vi "Demo File Dialog.vi"(8 "error in (no error)":errorcluster) -> (0 "error out":errorcluster)   [LabVIEW 2011]
uses:
  VIremote.llb/VIremoteEvent.ctl
  VIremote.llb/VIremoteFunction.ctl
panel:
  out "Selected File":path
  in  "Browse":bool
  in  "Select File":i32(ring)=1 items=["-C:\\_ics_ab\\dev\\vi.lib\\Throw Lab\\VIremote\\Examples", "Parent Folder", "-Folders", "server", "-Files", "All_Demos.vi", "Demo Accelerometer Graph.vi", "Demo Button and Alert server.vi", "Demo Button and Alert.vi", "Demo Combo Box.vi", "Demo Date and Time.vi", "Demo Dialog.vi", "Demo File Dialog.vi", "Demo Input Advanced.vi", "Demo Multitouch.vi", "Demo Navigation Bar More.vi", "Demo Navigation Bar.vi", "Demo Play wav file to Sound Output.vi", "Demo Ring and Enum.vi", "Demo Scrolling.vi", "Demo Simple Sound.vi", "Demo Slider.vi", "Demo Sound File to Sound Output.vi", "Demo Sound Input Output.vi", "Demo Sound Input.vi", "Demo Sound Input2.vi", "Demo String and Numeric.vi", "Demo UI Orientation.vi", "Demo User Notification and Status.vi", "Demo Video Input.vi", "Demo Video Input2.vi", "Hello World.vi", "sample.wav", "Server_Demo.vi", "VIremoteDisplaySimulator.vi", "VIs_for_All_Demos.vi", "xxx.vi"]
  in  "VIremoteEvent":T1=enum."Connection Closed"
  # "This is an example of how you could make a File Dialog. The ring above should be hidden under the button or the Selected File indicator. The code in the \"Ring Value Change\" case could be placed in a separate \"select path\" VI.\n\nThe Description of the ring above is:\n\nVIREMOTEPROPERTIES\nStyle=Grouped\nHeight=600\nUpdateWhileChanging\n\nThe height is for the iPad popover so it won't try to adjust its size. 600 is a good value for a large popover in both landscape and portrait mode.\n\nUpdateWhileChanging will prevent the table view to close when an item is selected."
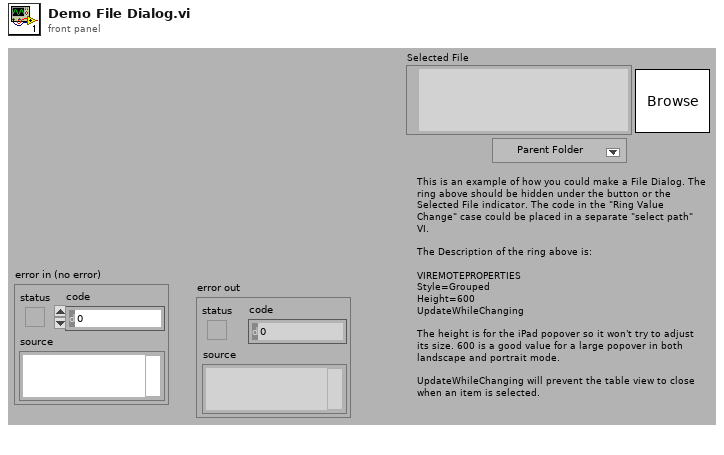
[diagram p1: front panel]
types:
  T1 = typedef "VIremoteEvent.ctl" = enum16{"No Event", "Connection Closed", "Navigate Back", "Enter Background", "Enter Foreground", "Portrait", "Portrait Upside Down", "Landscape Left", "Landscape Right"}
  T2 = typedef "VIremoteFunction.ctl" = enum16{"Do nothing", "Stop controller", "Close this connection", "Show info panel", "Set VI to control", "Set Accelerometer freq (Hz)", "Show Alert message", "Start Sound Input", "Stop Sound Input", "Set Volume (0-100)", "Set sound output Speaker", "Set sound output Receiver", "Play Sound", "Repeat Sound", "Stop Sound", "Pause Sound", "Resume Sound", "Set panel width of caller (320 or 480)", "Set Panel Size to Portrait", "Set Panel Size to Landscape", "Set Panel Size as Current Orientation", "Allow all UI Orientations", "Send user notification", "Disable Scrolling", "Normal Scrolling", "Page Scrolling", "Set Scroll Offset", "Page Indicator Position"}
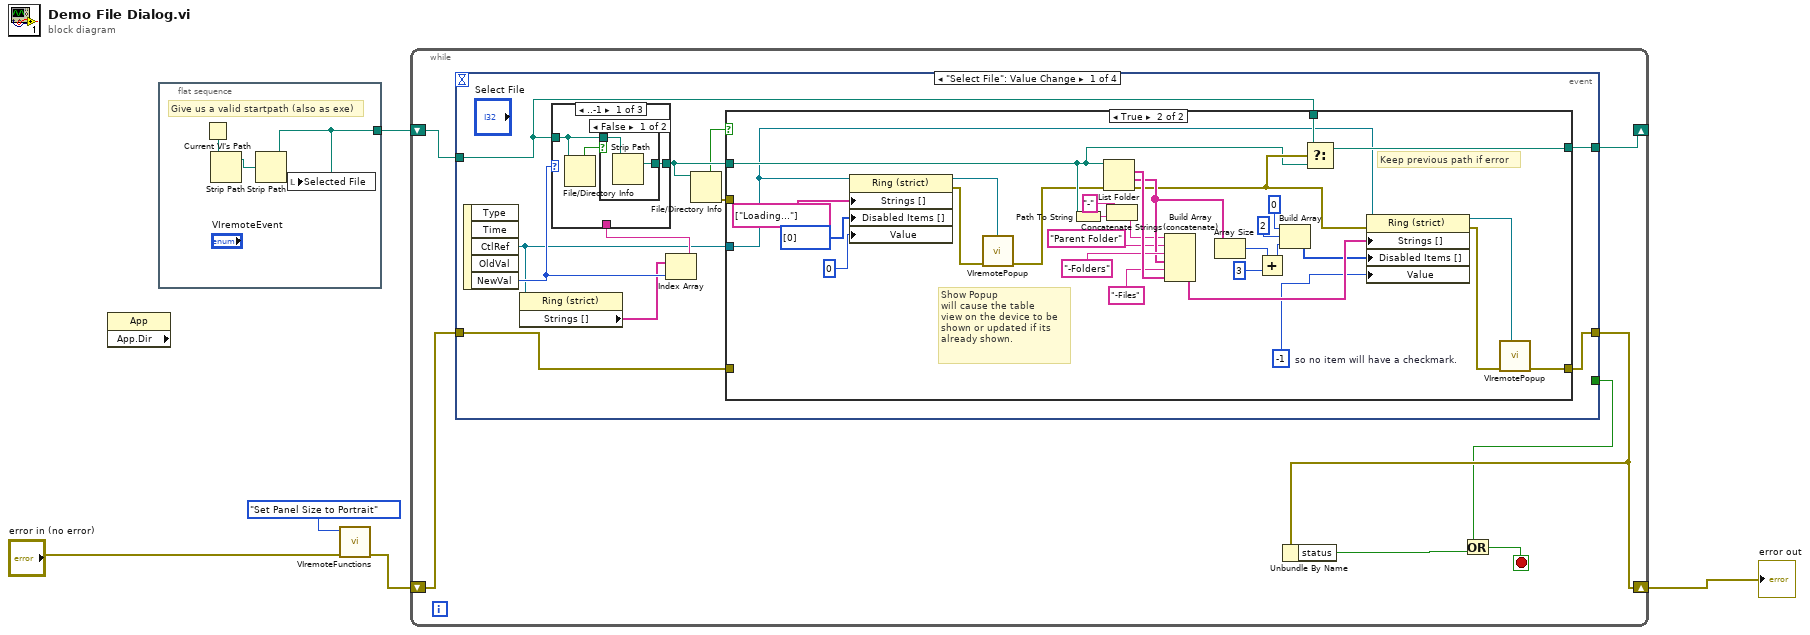
[diagram p0: block diagram]
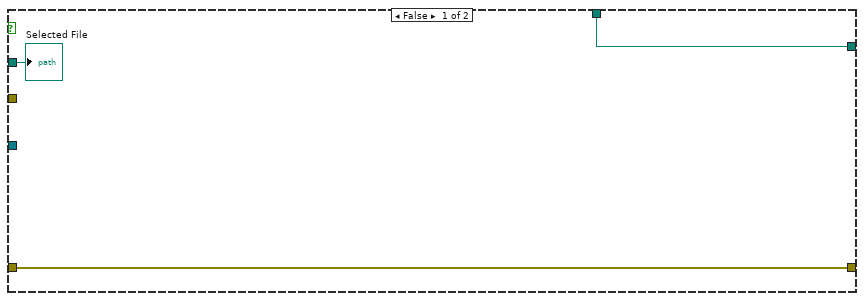
[diagram p2: hidden frame]
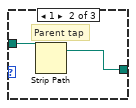
[diagram p4: hidden frame]
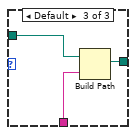
[diagram p5: hidden frame]
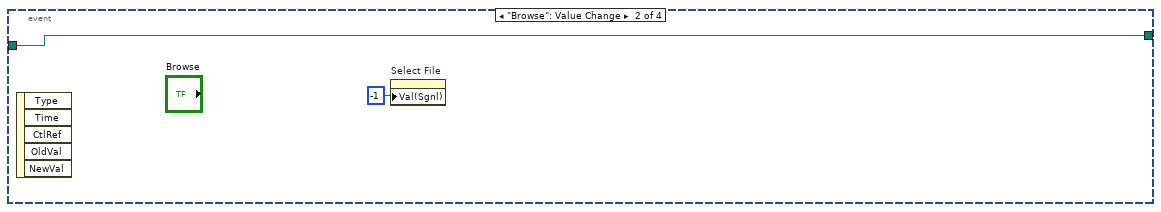
[diagram p6: hidden frame]
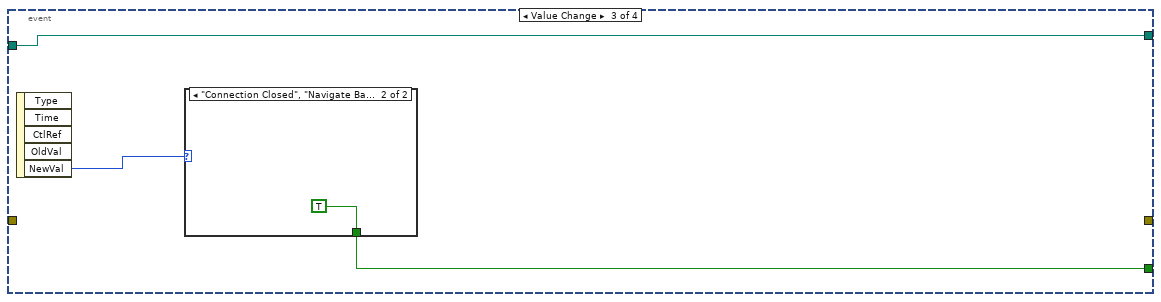
[diagram p7: hidden frame]
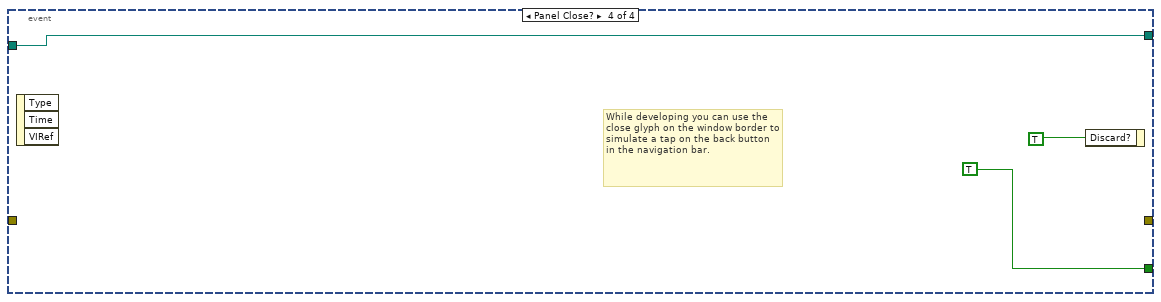
[diagram p9: hidden frame]
diagram:
  n1 = property class="App" props=["App.Dir"]() -> ()  [unwired: 2 in, 3 out]
  n2 = flat-sequence {
    tunnel: [w6] -> w1
    frame #0 {
      # "Give us a valid startpath (also as exe)"
      n3 = Current VI's Path() -> (path=w8:path)
      n4 = Strip Path(path=w8) -> (stripped path=w7:path)  [unwired: 1 out]
      n5 = Strip Path(path=w7) -> (stripped path=w6:path)  [unwired: 1 out]
      n6 = local write "Selected File"(w6) -> ()
    }
  }
  n7 = call "VIremoteFunctions.vi"("error in (no error)"="error in (no error)", "Function"=VIremoteFunction."Set Panel Size to Portrait") -> ("error out"=w4:errorcluster)  [unwired: 4 in, 5 out]
  n8 = while {
    shift-right: [w11] -> w2
    shift-left: w4 -> [w13]
    shift-right: [w14] -> _
    shift-left: w1 -> [w15]
    stop <- w9 stop-if-true
    n9 = event shown="[0] \"Select File\": Value Change" {
      selector: _ -> [_ _ _ _]
      dyn-events: _ -> [_ _ _ _]
      timeout: _ -> [_ _ _ _]
      tunnel: w15 -> [w24 w71 w75 w77]
      tunnel: [w23 w71 w75 w77] -> w14
      tunnel: w13 -> [w18 _ _ _]
      tunnel: [w19 _ _ _] -> w11
      tunnel: [_ _ w73 TRUE ("Discard?")] -> w10
      event "Select File": Value Change {
        n10 = event-data() -> ("CtlRef"=w17:refnum<vi>, "NewVal"=w25:i32)  [unwired: 4 out]
        n11 = property class="Ring (strict)"(reference=w17) -> ("Strings []"=w16:string[])  [unwired: 1 in, 2 out]
        n12 = Index Array(array=w16, index=w25) -> (element=w26:string)
        n13 = case shown="..-1" w25 {
          tunnel: w26 -> [_ _ w70]
          tunnel: [w61 w66 w69] -> w22
          tunnel: w24 -> [w60 w67 w68]
          frame ..-1 {
            n14 = File/Directory Info(path=w60) -> (directory=w62:bool)  [unwired: 1 in, 6 out]
            n15 = case shown="False" w62 {
              tunnel: [w64 w65] -> w61
              tunnel: w60 -> [w63 w65]
              frame False {
                n16 = Strip Path(path=w63) -> (stripped path=w64:path)  [unwired: 1 out]
              }
              frame True {
              }
            }
          }
          frame 1 {
            # "Parent tap"
            n17 = Strip Path(path=w67) -> (stripped path=w66:path)  [unwired: 1 out]
          }
          frame Default {
            n18 = Build Path(base path=w68, name or relative path=w70) -> (appended path=w69:path)
          }
        }
        n19 = File/Directory Info(path=w22) -> (directory=w21:bool, error out=w20:errorcluster)  [unwired: 1 in, 5 out]
        n20 = case shown="True" w21 {
          tunnel: w24 -> [w29 w52]
          tunnel: [w29 w51] -> w23
          tunnel: w22 -> [w27 w39]
          tunnel: w20 -> [_ _]
          tunnel: [w28 w48] -> w19
          tunnel: w18 -> [w28 _]
          tunnel: w17 -> [_ w34]
          frame False {
            "Selected File" <- w27
          }
          frame True {
            w41 = -1  # so no item will have a checkmark.
            # "Show Popup\nwill cause the table \nview on the device to be\nshown or updated if its\nalready shown."
            # "Keep previous path if error"
            n21 = property class="Ring (strict)"(reference=w34, "Strings []"=string[] ["Loading..."], "Disabled Items []"=i32[] [0], "Value"=0) -> (reference out=w31:refnum<vi>, error out=w33:errorcluster)  [unwired: 1 in]
            n22 = call "VIremotePopup.vi"("Control Refnum"=w31, "error in (no error)"=w33) -> ("error out"=w32:errorcluster)  [unwired: 1 in, 8 out]
            n23 = Path To String(path=w39) -> (string=w38:string)
            n24 = List Folder(path=w39, error in=w32) -> (filenames=w59:string[], folder names=w56:string[], error out=w44:errorcluster)  [unwired: 3 out]
            n25 = Concatenate Strings("-" ("string"), w38) -> (w36:string)
            n26 = Build Array (concatenate)(w36, "Parent Folder", "-Folders", w56, "-Files", w59) -> (w43:string[])
            n27 = Array Size(array=w56) -> (size(s)=w55:i32)
            n28 = Add(x=w55, y=3) -> (x+y=w50:i32)
            n29 = Build Array(0 ("y"), 2 ("y"), w50) -> (w42:i32[])
            n30 = Select(t=w52, s=w44, f=w39) -> (s? t:f=w51:path)
            n31 = property class="Ring (strict)"(reference=w34, error in=w44, "Strings []"=w43, "Disabled Items []"=w42, "Value"=w41) -> (reference out=w30:refnum<vi>, error out=w40:errorcluster)
            n32 = call "VIremotePopup.vi"("Control Refnum"=w30, "error in (no error)"=w40) -> ("error out"=w48:errorcluster)  [unwired: 1 in, 8 out]
          }
        }
      }
      event "Browse": Value Change {
        n33 = event-data() -> ()  [unwired: 6 out]
        n34 = property on="Select File" class="Ring (strict)"("Val(Sgnl)"=-1 ("Value (Signaling)")) -> ()  [unwired: 2 in, 2 out]
      }
      event Value Change {
        n35 = event-data() -> ("NewVal"=w74:T1)  [unwired: 5 out]
        n36 = case shown="\"Connection Closed\", \"Navigate Back\"" w74 {
          tunnel: [_ TRUE] -> w73
          frame "No Event", Default {
          }
          frame "Connection Closed", "Navigate Back" {
          }
        }
      }
      event Panel Close? {
        # "While developing you can use the close glyph on the window border to simulate a tap on the back button in the navigation bar."
        n37 = event-data() -> ()  [unwired: 4 out]
        n38 = event-data("Discard?"=TRUE) -> ()  [unwired: 1 in, 1 out]
      }
    }
    n39 = Unbundle By Name(w11) -> ("status"=w12:bool)
    n40 = Or(x=w10, y=w12) -> (x .or. y?=w9:bool)
  }
  "error out" <- w2
